vi "XNET Convert (Frame LIN to Byte Array).vi"(0 "session in":refnum<k21>, 5 "frame data":T1[](array[typedef]) {"event ID" format="%x"; "payload" format="%x"; "timestamp" format="%<%.7X\n%x>T"; "type" items=["LIN Data"=64, "LIN Bus Error"=65, "LIN No Response"=66, "Delay"=224, "Log Trigger"=225, "Start Trigger"=226]; "identifier" format="%x"}, 11 "error in (no error)":errorcluster) -> (4 "session out":refnum<k21>, 6 "signal data":u8[](array[numeric]), 15 "error out":errorcluster)   [LabVIEW 2018]
doc: "Converts NI-XNET LIN frame data to signal data."
uses:
  XNET Frame LIN.ctl
  XNET Frame Type LIN.ctl
  nixlvapi.dll
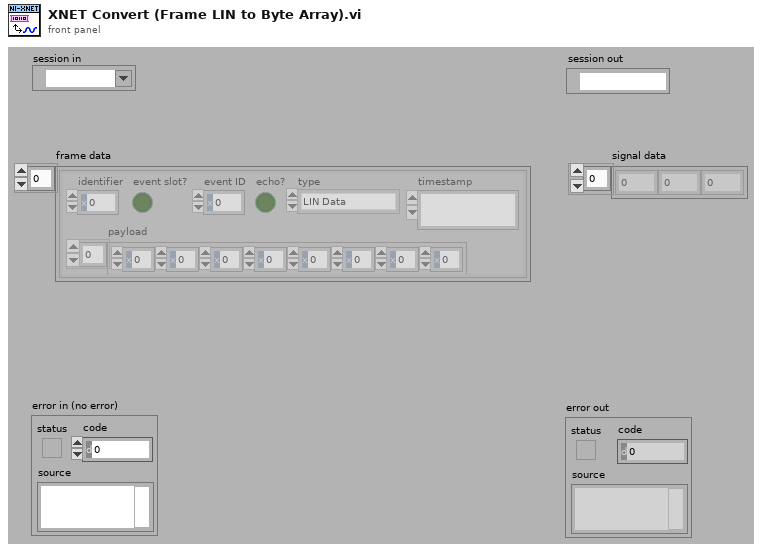
[diagram p1: front panel]
types:
  T1 = typedef "XNET Frame LIN.ctl" = cluster{"timestamp":timestamp, "payload":u8[], "identifier":u32, "type":T2, "event ID":u8, "event slot?":bool, "echo?":bool}
  T2 = typedef "XNET Frame Type LIN.ctl" = u8
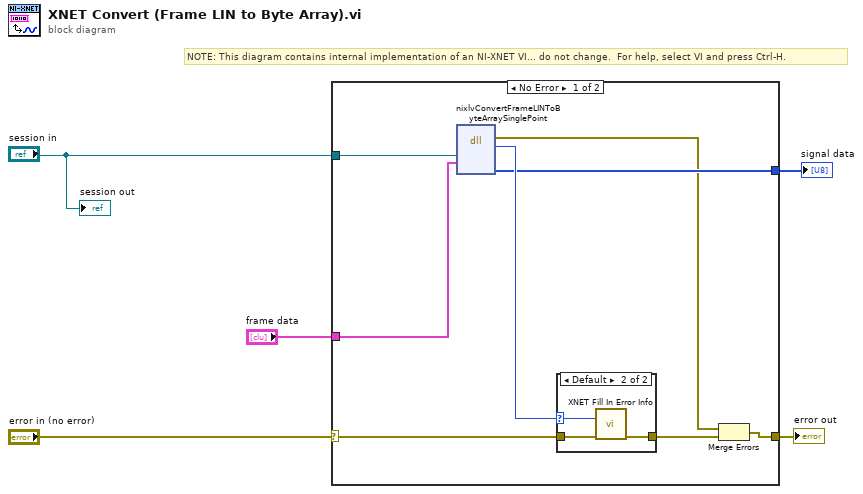
[diagram p0: block diagram]
diagram:
  # "NOTE: This diagram contains internal implementation of an NI-XNET VI... do not change.  For help, select VI and press Ctrl-H."
  n1 = case shown="No Error" "error in (no error)" {
    selector: "error in (no error)" -> [w12 w18]
    tunnel: "session in" -> [w13 _]
    tunnel: [w7 w18] -> w5
    tunnel: "frame data" -> [w9 _]
    tunnel: [w8 _] -> w2
    frame No Error {
      n2 = dll-call lib="nixlvapi.*" fn="nixlvConvertFrameLINToByteArraySinglePoint"("sessionRef"=w13, "frameData"=w9) -> (error out=w6:errorcluster, "return type"=w10:i32, "signalData"=w8:u8[])  [unwired: 4 in, 3 out]
      n3 = case shown="Default" w10 {
        selector: w10 -> [_ w15]
        tunnel: w12 -> [w14 w16]
        tunnel: [w14 w17] -> w11
        frame 0 {
        }
        frame Default {
          n4 = call "XNET Fill In Error Info.vi"("status code"=w15, "error in"=w16) -> ("error out"=w17:errorcluster)  [unwired: 13 out]
        }
      }
      n5 = Merge Errors(w6, w11) -> (w7:errorcluster)
    }
    frame Error {
    }
  }
  "error out" <- w5
  "signal data" <- w2
  "session out" <- "session in"
